vi "Arduino_ReadWrite.vi"() -> ()   [LabVIEW 2019]
uses:
  <vilib>/Utility/NIReport.llb/Report Type.ctl
  <vilib>/MakerHub/LINX/Public/Peripherals/Digital/Digital Read 1 Chan.vi
  <vilib>/MakerHub/LINX/Public/Peripherals/Digital/Digital Write 1 Chan.vi
  <vilib>/MakerHub/LINX/Public/Peripherals/Digital/Digital Read N Chans.vi
  <vilib>/MakerHub/LINX/Public/Peripherals/Digital/Digital Write N Chans.vi
  <vilib>/MakerHub/LINX/Private/Local IO/LinxDigitalRead.vi
  <vilib>/MakerHub/LINX/Public/Utilities/Check Channel.vi
  <vilib>/MakerHub/LINX/Private/Local IO/LinxDigitalWrite.vi
  <vilib>/MakerHub/LINX/Public/Utilities/Open Serial.vi
  <vilib>/MakerHub/LINX/Public/Sensors/Motion/Servo/Servo Open One Channel.vi
  <vilib>/Utility/NIReport.llb/Append Text Table to Report (wrap).vi
  <vilib>/MakerHub/LINX/Private/Utilties/Generate Error.vi
  <vilib>/MakerHub/LINX/Public/Sensors/Motion/Servo/Servo Set Pulse Width One Channel.vi
  <vilib>/MakerHub/LINX/Public/Sensors/Motion/Servo/Servo Close One Channel.vi
  <vilib>/Utility/NIReport.llb/NI_report.lvclass
  <vilib>/MakerHub/LINX/LMH-LINX.lvlib
  <vilib>/MakerHub/LINX/Public/Sensors/Distance/Ultrasonic/Ultrasonic.lvlib
  <vilib>/MakerHub/LINX/Public/Sensors/Motion/Servo/Servo.lvlib
  <vilib>/Analysis/NI_AALPro.lvlib
  <vilib>/Utility/NIReport.llb/Excel/NI_Excel.lvclass
  <vilib>/Utility/NIReport.llb/NI_ReportGenerationCore.lvlib
panel:
  out "Mesafe ve Fotosensör Veri Sayısı":i32
  out "Servo Motor Veri Sayısı":i32
  out "Servo Konum (0-180 Derece)":i64
  out "Servo Pozisyon Değişikliği":bool
  in  "Servo Motor Pozisyonları Kaydetme Yolu":path
  out "Buton Durum":i32
  out "Uyarı 2":string="Buton'a basılmıştır. Servo Motor'u kontrol etmeye başlayabilirsiniz."
  out "Servo Pozisyon Grafiği":dbl(graph)
  out "Buton Anlık":bool
  out "Alan Uyarı":string
  out "Mesafe Gösterge":string
  out "Uyarı":string
  out "Led Gösterge":bool
  out "Fotosensör (0-50) Gösterge":dbl(slide) scale=0.0..50.0
  in  "Fotonsensör Sınır Değeri":dbl
  out "Fotosensör (0-50)":dbl
  in  "Mesafe ve Fotosensör Verileri Kaydetme Yolu":path
  out "Mesafe Grafiği":dbl(graph)
  out "Mesafe":dbl
  in  "Stop Button":bool
  out "Loop Rate (Hz)":u32
  in  "Serial Port":refnum<visa-resource-name>
  # "Mesafe Sensörü ile Fotosensörden Verilerin Okunması Kaydedilmesi ve Servo Motor Kontrolü"
  # "Mesafe Sensöründen Verilerin Okunması ve Grafiği"
  # "Servo Motor Kontrolü ve Grafiği"
  # "Fotosensörden Verilerin Okunması ve Göstergesi"
  # "Verilerin Kaydedilmesi için Metin Dosyası Yolu Seçilmesi ve Veri Sayısı"
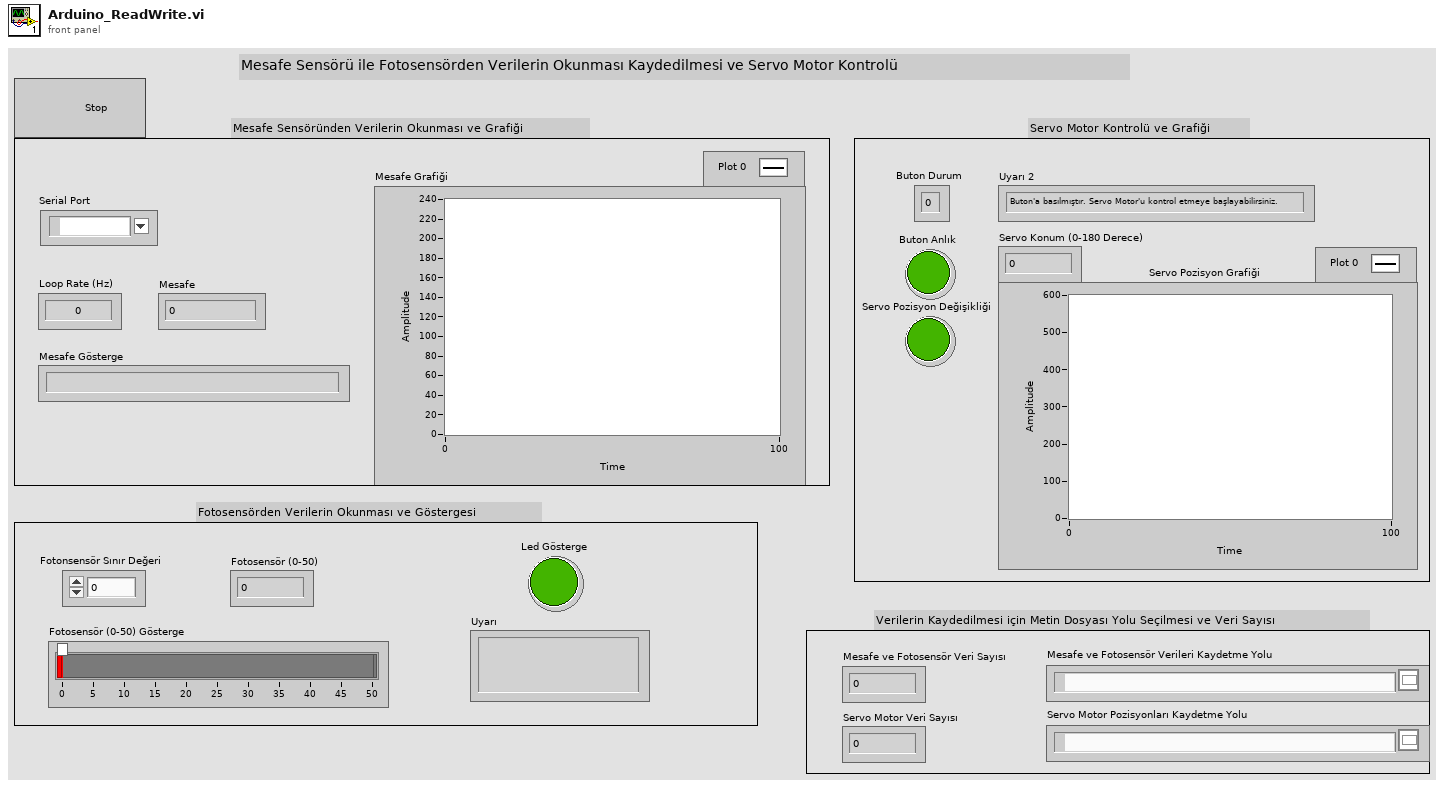
[diagram p1: front panel]
types:
  T1 = typedef "NI_ReportGenerationCore.lvlib/Report Type.ctl" = enum16{"HTML", "Word", "Excel"}
  T2 = enum16{"open", "replace", "create", "open or create", "replace or create", "replace or create with confirmation"}
  T3 = typedef "LMH-LINX.lvlib/LINX Ref.ctl" = cluster{"IO":T4, "Interface":T5, "LINX Device Config":T6}
  T4 = typedef "LMH-LINX.lvlib/Platform.ctl" = enum16{"Remote", "Local"}
  T5 = typedef "LMH-LINX.lvlib/Interface.ctl" = enum16{"Serial", "TCP"}
  T6 = typedef "LMH-LINX.lvlib/Device.lvlib/LINX Device Config.ctl" = cluster{"Interface":T5, "COM Port":refnum<visa-resource-name>, "TCP Configuration":T7, "Device Family":u8, "Device ID":u8, "Device Name":string, "TCP Ref":refnum<k5>, "Channels":T8}
  T7 = typedef "LMH-LINX.lvlib/Device.lvlib/TCP Config.ctl" = cluster{"IP Address":string, "Port":u16}
  T8 = typedef "LMH-LINX.lvlib/Channels.ctl" = cluster{"DI":u8[], "DO":u8[], "AI":u8[], "AO":u8[], "PWM":u8[], "QE":u8[], "UART":u8[], "I2C 2":u8[], "SPI":u8[], "CAN":u8[], "Servo":u8[], "AI Ref (V)":dbl, "AI Resolution (Bits)":u8, "AO Ref (V)":dbl, "AO Resolution (Bits)":u8}
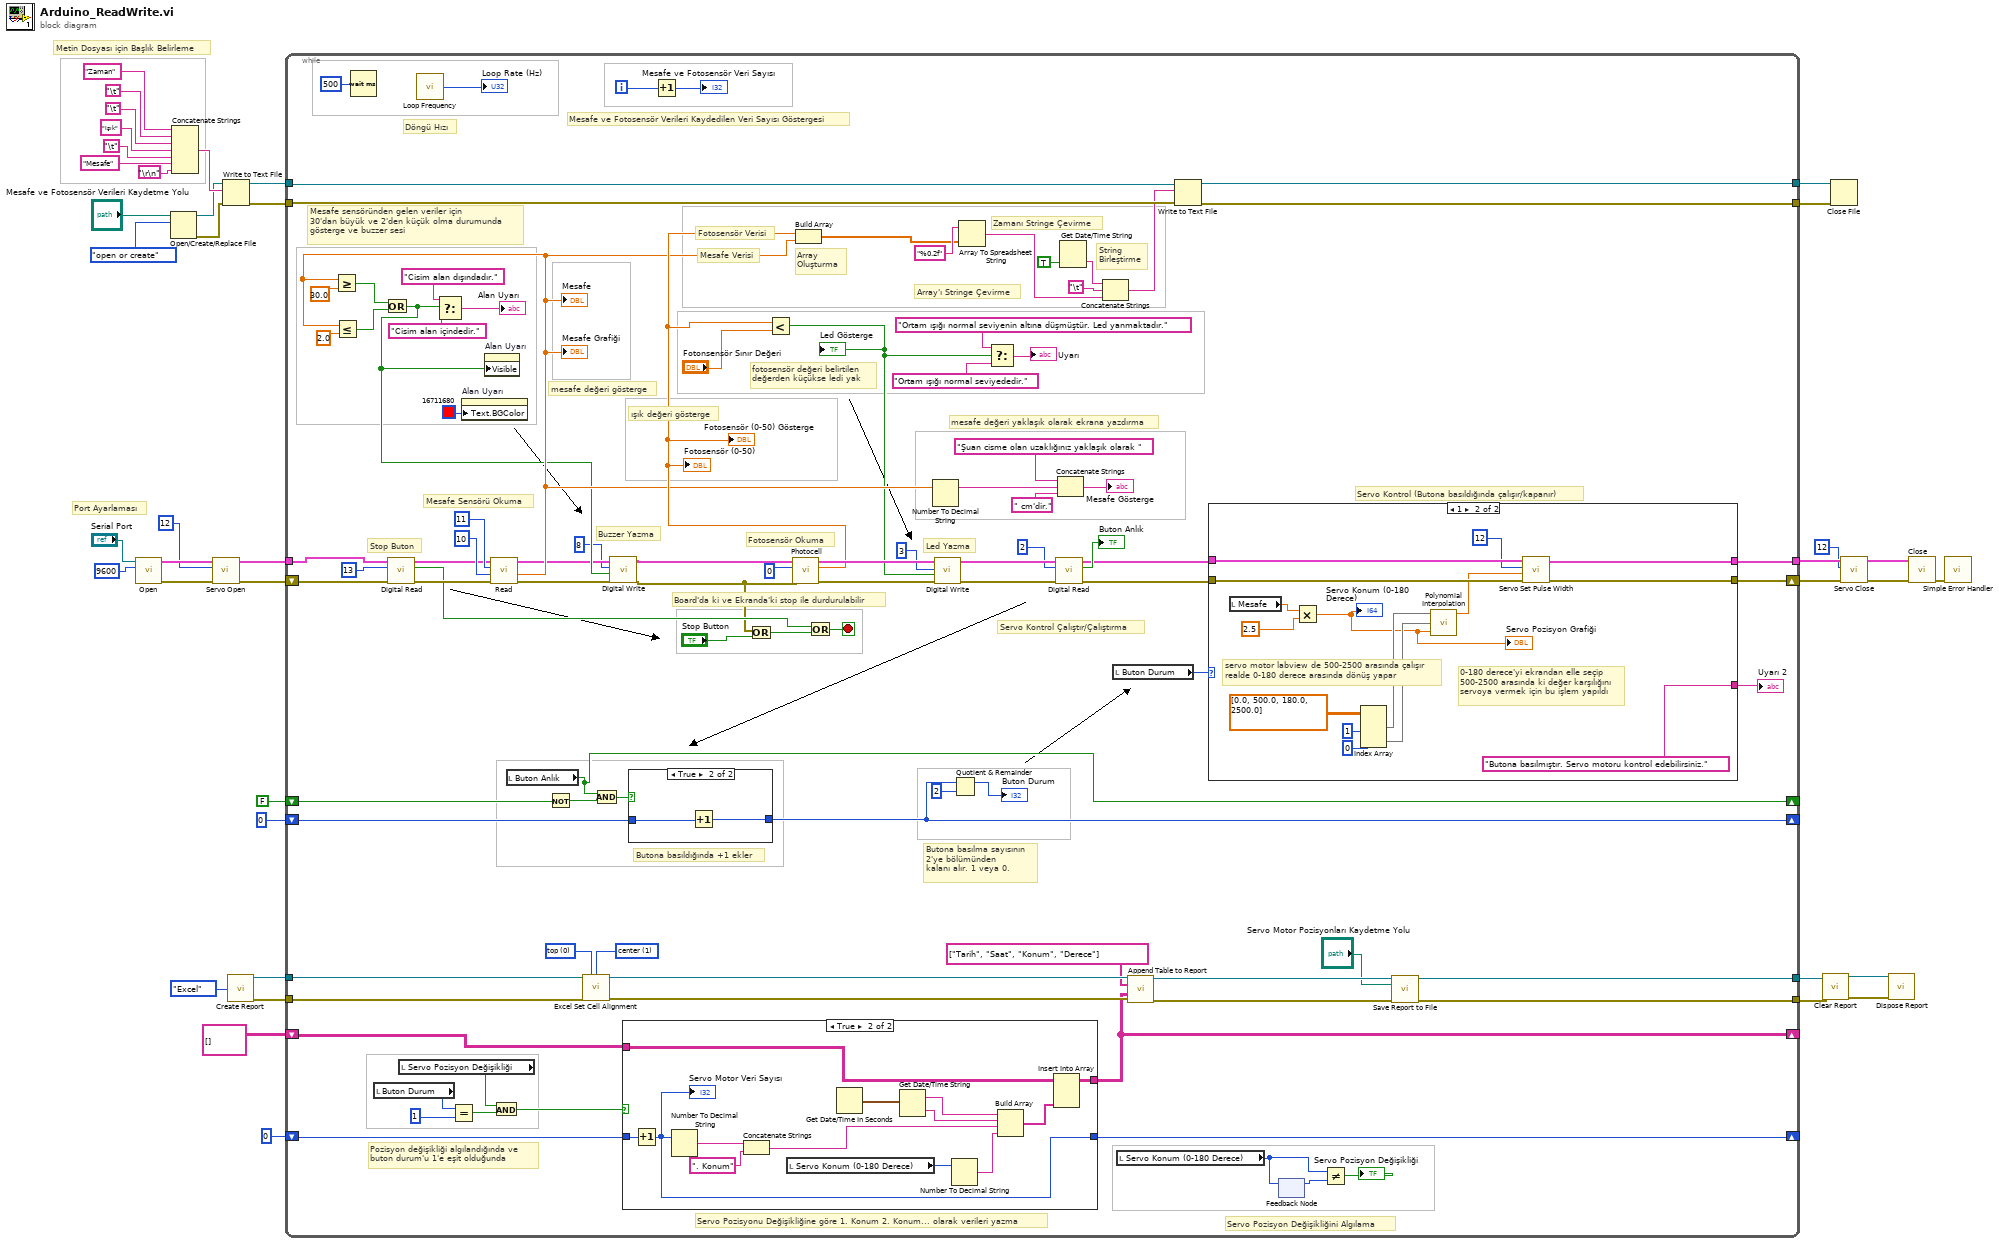
[diagram p0: block diagram]
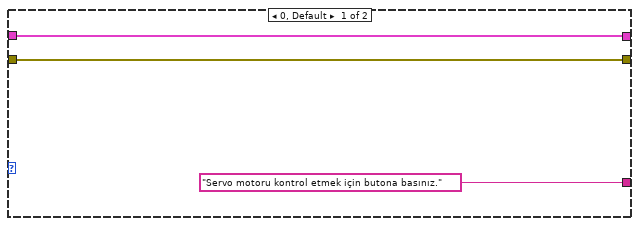
[diagram p4: hidden frame]
diagram:
  # "Metin Dosyası için Başlık Belirleme"
  # "Port Ayarlaması"
  n1 = call-poly <vilib>:"Open.vi"("Baud Rate Override"=u32 9600, "Serial Port"="Serial Port") -> ("Error Out"=w20:errorcluster, "LINX Resource"=w21:T3)  [unwired: 7 in, 1 out]
  n2 = Open/Create/Replace File(file path (use dialog)="Mesafe ve Fotosensör Verileri Kaydetme Yolu", operation (0:open)=T2."open or create") -> (refnum out=w28:refnum<file>, error out=w27:errorcluster)  [unwired: 4 in, 1 out]
  n3 = Concatenate Strings("Zaman" ("string"), "\t", "\t", "Işık" ("string"), "\t", "Mesafe" ("string"), "\r\n") -> (w29:string)
  n4 = call-poly <vilib>:"Servo Open.vi"("Error In"=w20, "Servo Channel"=u8 12, "LINX Resource"=w21) -> ("Error Out"=w18:errorcluster, "LINX Resource"=w19:T3)  [unwired: 7 in]
  n5 = Write to Text File(file (use dialog)=w28, text=w29, error in=w27) -> (refnum out=w33:refnum<file>, error out=w32:errorcluster)  [unwired: 1 in, 1 out]
  n6 = call <vilib>:"Create Report.vi"("report type"=Report_Type."Excel") -> ("report out"=w8:refnum<class "NI_report.lvclass">, "error out"=w7:errorcluster)  [unwired: 13 in]
  n7 = while {
    tunnel: w19 -> [w129]
    tunnel: [w78] -> w16
    shift-right: [w77] -> w15
    shift-left: w18 -> [w131]
    tunnel: w33 -> [w105]
    tunnel: w32 -> [w107]
    tunnel: [w104] -> w35
    tunnel: [w106] -> w34
    shift-right: [w68] -> _
    shift-left: FALSE -> [w73]
    shift-right: [w69] -> _
    shift-left: 0 -> [w72]
    tunnel: w8 -> [w51]
    tunnel: w7 -> [w50]
    tunnel: [w49] -> w4
    tunnel: [w48] -> w3
    shift-right: [w45] -> _
    shift-left: string[][] [] -> [w47]
    shift-right: [w44] -> _
    shift-left: 0 -> [w46]
    i -> [w42]
    stop <- w125 stop-if-true
    w66 = 1 items=["left", "center", "right"] ("horizontal alignment (left)")
    w67 = 0 items=["top", "center", "bottom"] ("vertical alignment (top)")
    # "Pozisyon değişikliği algılandığında ve\nbuton durum'u 1'e eşit olduğunda"
    # "Servo Pozisyonu Değişikliğine göre 1. Konum 2. Konum... olarak verileri yazma"
    # "Servo Pozisyon Değişikliğini Algılama"
    # "Butona basılma sayısının\n2'ye bölümünden\nkalanı alır. 1 veya 0."
    # "Butona basıldığında +1 ekler"
    # "Servo Kontrol (Butona basıldığında çalışır/kapanır)"
    # "Servo Kontrol Çalıştır/Çalıştırma"
    # "Board'da ki ve Ekranda'ki stop ile durdurulabilir"
    # "mesafe değeri yaklaşık olarak ekrana yazdırma"
    # "mesafe değeri gösterge"
    # "Mesafe sensöründen gelen veriler için \n30'dan büyük ve 2'den küçük olma durumunda\ngösterge ve buzzer sesi"
    # "Mesafe ve Fotosensör Verileri Kaydedilen Veri Sayısı Göstergesi"
    # "Buzzer Yazma"
    # "Fotosensör Okuma"
    # "Led Yazma"
    # "String \nBirleştirme"
    # "Zamanı Stringe Çevirme"
    # "Array'ı Stringe Çevirme"
    # "Fotosensör Verisi"
    # "Mesafe Verisi"
    # "Array \nOluşturma"
    # "ışık değeri gösterge"
    # "fotosensör değeri belirtilen \ndeğerden küçükse ledi yak"
    # "Stop Buton"
    # "Döngü Hızı"
    # "Mesafe Sensörü Okuma"
    n8 = Wait (ms)(milliseconds to wait=u32 500) -> ()  [unwired: 1 out]
    n9 = local read "Buton Durum"() -> (w52:i32)
    n10 = call-poly <vilib>:"Digital Read.vi"("Error In"=w131, "DI Channel"=u8 13, "LINX Resource"=w129) -> ("Error Out"=w130:errorcluster, "DI Value"=w127:bool, "LINX Resource"=w128:T3)  [unwired: 6 in]
    n11 = local read "Servo Pozisyon Değişikliği"() -> (w56:bool)
    n12 = call <vilib>:"Loop Frequency.vi"() -> ("Loop Rate (Hz)"=→"Loop Rate (Hz)":u32)
    n13 = Equal?(x=w52, y=1) -> (x = y?=w55:bool)
    n14 = property on="Alan Uyarı" class="Str"("Text.BGColor"=u32 16711680 ("Text.Text Colors:BG Color")) -> ()  [unwired: 2 in, 2 out]
    n15 = call <vilib>:"Read.vi"("Error In"=w130, "DO Channel"=u8 10, "DI Channel"=u8 11, "LINX Resource"=w128) -> ("Error Out"=w88:errorcluster, "Centimeters"=w93:dbl, "LINX Resource"=w90:T3)  [unwired: 4 in, 1 out]
    "Mesafe" <- w93
    "Mesafe Grafiği" <- w93
    n16 = Greater Or Equal?(x=w93, y=30.0) -> (x >= y?=w98:bool)
    n17 = Less Or Equal?(x=w93, y=2.0) -> (x <= y?=w97:bool)
    n18 = Or(x=w98, y=w97) -> (x .or. y?=w91:bool)
    n19 = Select(t="Cisim alan dışındadır.", s=w91, f="Cisim alan içindedir.") -> (s? t:f=→"Alan Uyarı":string)
    n20 = property on="Alan Uyarı" class="Str"("Visible"=w91) -> ()  [unwired: 2 in, 2 out]
    n21 = And(x=w56, y=w55) -> (x .and. y?=w54:bool)
    n22 = local read "Buton Anlık"() -> (w68:bool)
    n23 = Not(x=w73) -> (.not. x?=w75:bool)
    n24 = call <vilib>:"Excel Set Cell Alignment.vi"("report in"=w51, "vertical alignment (top)"=w67, "horizontal alignment (left)"=w66, "error in (no error)"=w50) -> ("report out"=w65:refnum<class "NI_report.lvclass">, "error out"=w64:errorcluster)  [unwired: 10 in]
    n25 = And(x=w68, y=w75) -> (x .and. y?=w74:bool)
    n26 = call-poly <vilib>:"Digital Write.vi"("Error In"=w88, "Output Value"=w91, "DO Channel"=u8 8, "LINX Resource"=w90) -> ("Error Out"=w86:errorcluster, "LINX Resource"=w89:T3)  [unwired: 6 in]
    n27 = case shown="True" w54 {
      tunnel: [w139 w144] -> w45
      tunnel: w47 -> [w139 w143]
      tunnel: w46 -> [w138 w142]
      tunnel: [w138 w141] -> w44
      frame False {
      }
      frame True {
        n28 = Increment(x=w142) -> (x+1=w141:i32)
        "Servo Motor Veri Sayısı" <- w141
        n29 = Number To Decimal String(number=w141) -> (decimal integer string=w149:string)  [unwired: 1 in]
        n30 = Concatenate Strings(w149, ". Konum" ("string")) -> (w150:string)
        n31 = local read "Servo Konum (0-180 Derece)"() -> (w140:i64)
        n32 = Get Date/Time In Seconds() -> (seconds since 1Jan1904=w146:timestamp)
        n33 = Get Date/Time String(seconds (now)=w146) -> (date string=w147:string, time string=w148:string)  [unwired: 2 in]
        n34 = Number To Decimal String(number=w140) -> (decimal integer string=w151:string)  [unwired: 1 in]
        n35 = Build Array(w147, w148, w150, w151) -> (w152:string[])
        n36 = Insert Into Array(array=w143, new element=w152) -> (w144:string[][])  [unwired: 2 in]
      }
    }
    n37 = case shown="True" w74 {
      tunnel: w72 -> [w153 w155]
      tunnel: [w153 w154] -> w69
      frame False {
      }
      frame True {
        n38 = Increment(x=w155) -> (x+1=w154:i32)
      }
    }
    n39 = Increment(x=w42) -> (x+1=→"Mesafe ve Fotosensör Veri Sayısı":i32)
    n40 = Or(x=w86, y="Stop Button") -> (x .or. y?=w126:bool)
    n41 = call <vilib>:"Photocell.vi"("Error In"=w86, "AI Channel"=u8 0, "LINX Resource"=w89) -> ("Error Out"=w119:errorcluster, "Value (0-100)"=w114:dbl, "LINX Resource"=w120:T3)  [unwired: 6 in]
    "Fotosensör (0-50)" <- w114
    "Fotosensör (0-50) Gösterge" <- w114
    n42 = Less?(x=w114, y="Fotonsensör Sınır Değeri") -> (x < y?=w85:bool)
    "Led Gösterge" <- w85
    n43 = Build Array(w114, w93) -> (w112:dbl[])
    n44 = Or(x=w127, y=w126) -> (x .or. y?=w125:bool)
    n45 = Number To Decimal String(number=w93) -> (decimal integer string=w124:string)  [unwired: 1 in]
    n46 = call-poly <vilib>:"Digital Write.vi"("Error In"=w119, "Output Value"=w85, "DO Channel"=u8 3, "LINX Resource"=w120) -> ("Error Out"=w83:errorcluster, "LINX Resource"=w84:T3)  [unwired: 6 in]
    n47 = Quotient & Remainder(x=w69, y=2) -> (x-y*floor(x/y)=→"Buton Durum":i32)  [unwired: 1 out]
    n48 = Array To Spreadsheet String(array=w112, 3:"%0.2f" ("format string")) -> (spreadsheet string=w108:string)  [unwired: 1 in]
    n49 = Select(t="Ortam ışığı normal seviyenin altına düşmüştür. Led yanmaktadır.", s=w85, f="Ortam ışığı normal seviyededir.") -> (s? t:f=→"Uyarı":string)
    n50 = call-poly <vilib>:"Digital Read.vi"("Error In"=w83, "DI Channel"=u8 2, "LINX Resource"=w84) -> ("Error Out"=w79:errorcluster, "DI Value"=→"Buton Anlık":bool, "LINX Resource"=w80:T3)  [unwired: 6 in]
    n51 = Concatenate Strings("Şuan cisme olan uzaklığınız yaklaşık olarak " ("string"), w124, " cm'dir." ("string")) -> (→"Mesafe Gösterge":string)
    n52 = Get Date/Time String(want seconds? (F)=TRUE) -> (time string=w109:string)  [unwired: 2 in, 1 out]
    n53 = Concatenate Strings(w109, "\t", w108) -> (w103:string)
    n54 = local read "Buton Durum"() -> (w43:i32)
    n55 = local read "Servo Konum (0-180 Derece)"() -> (w58:i64)
    n56 = call-poly <vilib>:"Append Table to Report.vi"("report in"=w65, "column headers"=string[] ["Tarih", "Saat", "Konum", "Derece"], "text data"=w45, "error in (no error)"=w64) -> ("report out"=w63:refnum<class "NI_report.lvclass">, "error out"=w62:errorcluster)  [unwired: 8 in, 2 out]
    n57 = Write to Text File(file (use dialog)=w105, text=w103, error in=w107) -> (refnum out=w104:refnum<file>, error out=w106:errorcluster)  [unwired: 1 in, 1 out]
    n58 = case shown="1" w43 {
      tunnel: [w157 w173] -> w77
      tunnel: [w158 w172] -> w78
      tunnel: w80 -> [w158 w171]
      tunnel: w79 -> [w157 w170]
      tunnel: ["Servo motoru kontrol etmek için butona basınız." "Butona basılmıştır. Servo motoru kontrol edebilirsiniz."] -> w76
      frame 0, Default {
      }
      frame 1 {
        # "0-180 derece'yi ekrandan elle seçip\n500-2500 arasında ki değer karşılığını\nservoya vermek için bu işlem yapıldı"
        # "servo motor labview de 500-2500 arasında çalışır\nrealde 0-180 derece arasında dönüş yapar"
        n59 = local read "Mesafe"() -> (w160:dbl)
        n60 = Multiply(x=w160, y=2.5) -> (x*y=w159:dbl)
        "Servo Pozisyon Grafiği" <- w159
        "Servo Konum (0-180 Derece)" <- w159
        n61 = Index Array(array=dbl[][] [[0.0, 500.0], [180.0, 2500.0]], index (col) #1=1 ("disabled index (col)"), index (col) #2=0 ("index (col)")) -> (element #1=w167:dbl[], element #2=w166:dbl[])  [unwired: 2 in]
        n62 = call <vilib>:"Polynomial Interpolation.vi"("x value"=w159, "X"=w166, "Y"=w167) -> ("interpolation value"=w163:dbl)  [unwired: 2 out]
        n63 = call-poly <vilib>:"Servo Set Pulse Width.vi"("Error In"=w170, "Pulse Width (uS)"=w163, "Servo Channel"=u8 12, "LINX Resource"=w171) -> ("Error Out"=w173:errorcluster, "LINX Resource"=w172:T3)  [unwired: 6 in]
      }
    }
    "Uyarı 2" <- w76
    n64 = feedback #1() -> (w59:i64)  [unwired: 1 in]
    n65 = feedback-in #1(w58) -> ()
    n66 = Not Equal?(x=w58, y=w59) -> (x != y?=→"Servo Pozisyon Değişikliği":bool)
    n67 = call-dynamic "Save Report to File.vi"("report in"=w63, "report file path"="Servo Motor Pozisyonları Kaydetme Yolu", "error in (no error)"=w62) -> ("report out"=w49:refnum<class "NI_report.lvclass">, "error out"=w48:errorcluster)  [unwired: 11 in]
  }
  n68 = call-dynamic "Clear Report.vi"("report in"=w4, "error in (no error)"=w3) -> ("report out"=w6:refnum<class "NI_report.lvclass">, "error out"=w5:errorcluster)  [unwired: 12 in]
  n69 = Close File(refnum=w35, error in=w34) -> ()  [unwired: 2 out]
  n70 = call-poly <vilib>:"Servo Close.vi"("Error In"=w15, "Servo Channel"=u8 12, "LINX Resource"=w16) -> ("Error Out"=w13:errorcluster, "LINX Resource"=w14:T3)  [unwired: 7 in]
  n71 = call-dynamic "Dispose Report.vi"("report in"=w6, "error in (no error)"=w5) -> ()  [unwired: 13 in, 1 out]
  n72 = call <vilib>:"Close.vi"("Error In"=w13, "LINX Resource"=w14) -> ("Error Out"=w39:errorcluster)  [unwired: 9 in]
  n73 = call <vilib>:"Simple Error Handler.vi"("error in (no error)"=w39) -> ()  [unwired: 4 in, 5 out]
